vi "Compare Folder Shots.vi"(8 "error in (no error)":errorcluster, 10 "Folder Shot 2":T2[](array[typedef]), 11 "Folder Shot 1":T2[](array[typedef])) -> (0 "error out":errorcluster, 3 "Folder Shot Results":T1)   [LabVIEW 2016, in "SLL File IO.lvlib"]
doc: "Compare two Folder Shot Clusters."
uses:
  SLL File IO.lvlib
  _Typedefs/Folder Shot Element.ctl
  _Typedefs/Folder Shot Result.ctl
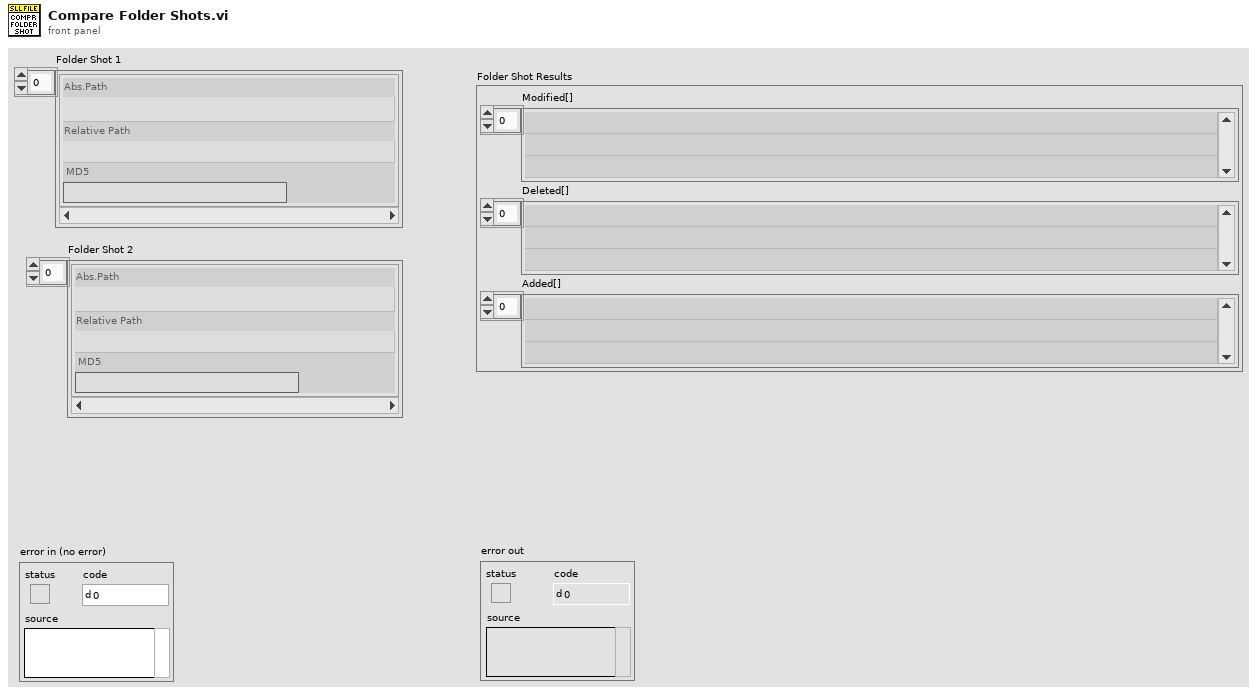
[diagram p1: front panel]
types:
  T1 = typedef "SLL File IO.lvlib/Folder Shot Result.ctl" = cluster{"Modified[]":path[], "Deleted[]":path[], "Added[]":path[]}
  T2 = typedef "SLL File IO.lvlib/Folder Shot Element.ctl" = cluster{"Abs.Path":path, "Relative Path":path, "MD5":string}
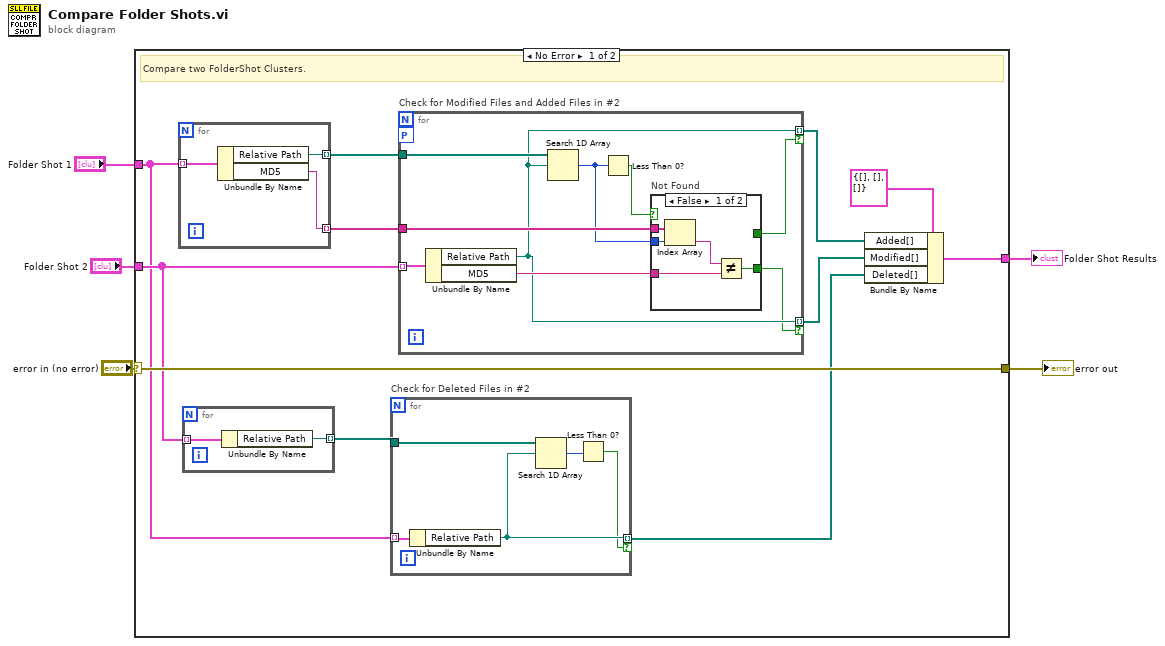
[diagram p0: block diagram]
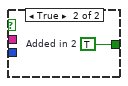
[diagram p2: hidden frame]
diagram:
  n1 = case shown="No Error" "error in (no error)" {
    selector: "error in (no error)" -> [w16 w42]
    tunnel: [w16 w42] -> w4
    tunnel: "Folder Shot 1" -> [w12 _]
    tunnel: "Folder Shot 2" -> [w13 _]
    tunnel: [w6 _] -> w1
    frame No Error {
      # "Compare two FolderShot Clusters."
      n2 = for {
        tunnel: w12 -> [w41] mode=indexing
        tunnel: [w40] -> w15 mode=indexing
        tunnel: [w39] -> w14 mode=indexing
        n3 = Unbundle By Name(w41) -> ("Relative Path"=w40:path, "MD5"=w39:string)
      }
      n4 = for {
        tunnel: w13 -> [w23] mode=indexing
        tunnel: [w22] -> w11 mode=indexing
        n5 = Unbundle By Name(w23) -> ("Relative Path"=w22:path)
      }
      n6 = for "Check for Deleted Files in #2" {
        tunnel: w12 -> [w20] mode=indexing
        tunnel: w11 -> [w21]
        tunnel: [w18] -> w7 mode=indexing if=w17
        n7 = Unbundle By Name(w20) -> ("Relative Path"=w18:path)
        n8 = Search 1D Array(1D array=w21, element=w18) -> (index of element=w19:i32)  [unwired: 1 in]
        n9 = Less Than 0?(x=w19) -> (x < 0?=w17:bool)
      }
      n10 = for "Check for Modified Files and Added Files in #2" {
        tunnel: w13 -> [w32] mode=indexing
        tunnel: w15 -> [w31]
        tunnel: w14 -> [w30]
        tunnel: [w26] -> w9 mode=indexing if=w24
        tunnel: [w26] -> w8 mode=indexing if=w25
        workers-P: _ -> [_]
        n11 = Unbundle By Name(w32) -> ("Relative Path"=w26:path, "MD5"=w29:string)
        n12 = Search 1D Array(1D array=w31, element=w26) -> (index of element=w28:i32)  [unwired: 1 in]
        n13 = Less Than 0?(x=w28) -> (x < 0?=w27:bool)
        n14 = case "Not Found" shown="False" w27 {
          tunnel: w30 -> [w37 _]
          tunnel: w29 -> [w35 _]
          tunnel: w28 -> [w34 _]
          tunnel: [w33 _] -> w25
          tunnel: [_ w38] -> w24
          frame False {
            n15 = Index Array(array=w37, index=w34) -> (element=w36:string)
            n16 = Not Equal?(x=w36, y=w35) -> (x != y?=w33:bool)
          }
          frame True {
            w38 = TRUE  # Added in 2
          }
        }
      }
      n17 = Bundle By Name(cluster=T1 {"Modified[]"=[], "Deleted[]"=[], "Added[]"=[]} ("Folder Shot Results"), "Added[]"=w9, "Modified[]"=w8, "Deleted[]"=w7) -> (w6:T1)
    }
    frame Error {
    }
  }
  "error out" <- w4
  "Folder Shot Results" <- w1
